vi "Set IO Pulse Data.vi"(8 "error in (no error)":errorcluster, 9 "duty":dbl, 10 "hz":dbl, 11 "channel":u8) -> (0 "error out":errorcluster)   [LabVIEW 2021, in "vmmso.lvlib"]
doc: "DLL_API void WINAPI SetIOPulseData(unsigned char channel, double hz, double duty);"
uses:
  vmmso.lvlib
  vmmso.dll
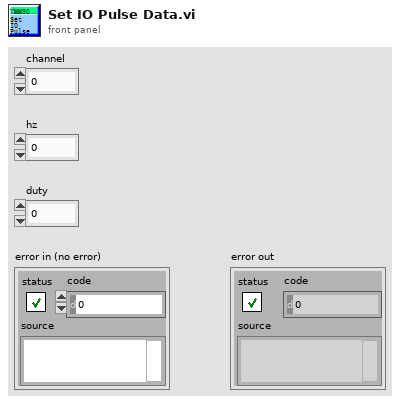
[diagram p1: front panel]
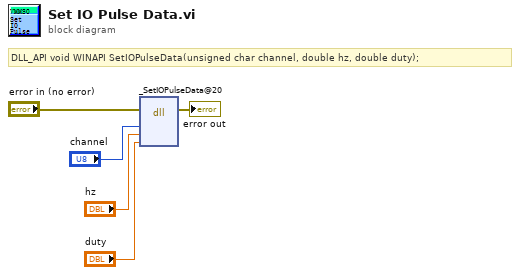
[diagram p0: block diagram]
diagram:
  # "DLL_API void WINAPI SetIOPulseData(unsigned char channel, double hz, double duty);"
  n1 = dll-call lib="O:/MSO/library/demo-Labview/vmmso/vmmso.*" fn="_SetIOPulseData@20"(error in="error in (no error)", "channel"="channel", "hz"="hz", "duty"="duty") -> (error out=→"error out":errorcluster)  [unwired: 6 in, 1 out]
